vi "Generate Shadow State JSON.vi"(11 "State":T1[](array[typedef])) -> (3 "JSON":string)   [LabVIEW 2015, in "NI_AWS_IoT.lvlib"]
uses:
  NI_AWS_IoT.lvlib
  JSON Parsing/Name-Value with Type.ctl
  JSON Parsing/Name Value Pair.ctl
  JSON Parsing/JSON Type.ctl
  JSON Parsing/NI_JSON Parsing.lvlib
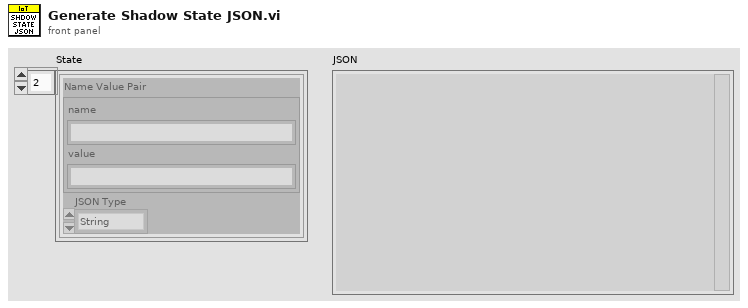
[diagram p1: front panel]
types:
  T1 = typedef "NI_JSON Parsing.lvlib/Name-Value with Type.ctl" = cluster{"Name Value Pair":T2, "JSON Type":T3}
  T2 = typedef "NI_JSON Parsing.lvlib/Name Value Pair.ctl" = cluster{"name":string, "value":string}
  T3 = typedef "NI_JSON Parsing.lvlib/JSON Type.ctl" = enum16{"String", "Numeric", "Boolean"}
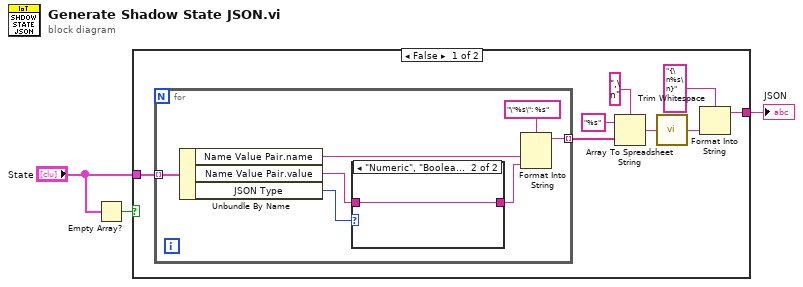
[diagram p0: block diagram]
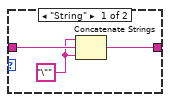
[diagram p2: hidden frame]
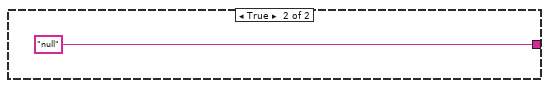
[diagram p3: hidden frame]
diagram:
  n1 = Empty Array?(array="State") -> (empty?=w3:bool)
  n2 = case shown="False" w3 {
    tunnel: "State" -> [w11 _]
    tunnel: [w4 "null"] -> w1
    frame False {
      n3 = for {
        tunnel: w11 -> [w18] mode=indexing
        tunnel: [w12] -> w10 mode=indexing
        n4 = Unbundle By Name(w18) -> ("Name Value Pair.name"=w16:string, "Name Value Pair.value"=w14:string, "JSON Type"=w15:T3)
        n5 = case shown="\"Numeric\", \"Boolean\"" w15 {
          tunnel: w14 -> [w21 w22]
          tunnel: [w20 w22] -> w13
          frame "String" {
            w19 = "\""
            n6 = Concatenate Strings(w19, w21, w19) -> (w20:string)
          }
          frame "Numeric", "Boolean" {
          }
        }
        n7 = Format Into String(format string="\"%s\": %s", w16, w13) -> (resulting string=w12:string)  [unwired: 2 in, 1 out]
      }
      n8 = Array To Spreadsheet String(delimiter (Tab)=",\n", array=w10, 3:"%s" ("format string")) -> (spreadsheet string=w7:string)
      n9 = call <vilib>:"Trim Whitespace.vi"("string"=w7) -> ("trimmed string"=w6:string)  [unwired: 1 in]
      n10 = Format Into String(format string="{\n%s\n}", w6) -> (resulting string=w4:string)  [unwired: 2 in, 1 out]
    }
    frame True {
    }
  }
  "JSON" <- w1
